vi "Line follower Color Stop.vi"(6 "Target reflection":sgl=25.0, 7 "Threshold to Color":i32=1200, 8 "Threshold to slow":i32=1000, 9 "Min. speed":i32=20, 10 "Max. speed":i32=40, 11 "EV3 in":T1) -> (3 "EV3 out":T1)   [LabVIEW 2016]
uses:
  <vilib>/NXT/Subs/LVHSConnector.ctl
  <vilib>/NXT/LegoClasses/BrickReference/BrickReference.lvclass
  <vilib>/NXT/Block Support/NXT_OutputPort.ctl
  <vilib>/NXT/Block Support/NXT_InputPort.ctl
  <vilib>/NXT/NXTIO Xnodes/NXTIONodeSubVIs/LEGOResetMotors.vi
  <vilib>/NXT/Dual Mode Library/Motors/Rotation.vi
  <vilib>/NXT/Dual Mode Library/Sensors/EV3_Color_Reflect.vi
  <vilib>/NXT/NXTIO Xnodes/NXTIONodeSubVIs/NXTMotorSteeringOn.vi
  <vilib>/NXT/NXTIO Xnodes/NXTIONodeSubVIs/NXTStopMotors.vi
  <vilib>/NXT/Dual Mode Library/Waits/Wait_Num.vi
  <vilib>/NXT/NXTIO Xnodes/NXTIOXNode/NXTIO.xnode
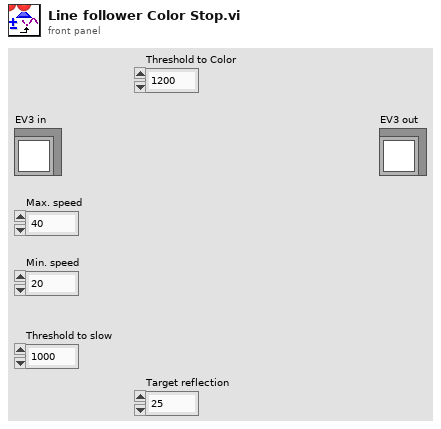
[diagram p1: front panel]
types:
  T1 = typedef "LVHSConnector.ctl" = refnum<class "BrickReference.lvclass">
  T2 = typedef "NXT_OutputPort.ctl" = u8
  T3 = typedef "NXT_InputPort.ctl" = u32
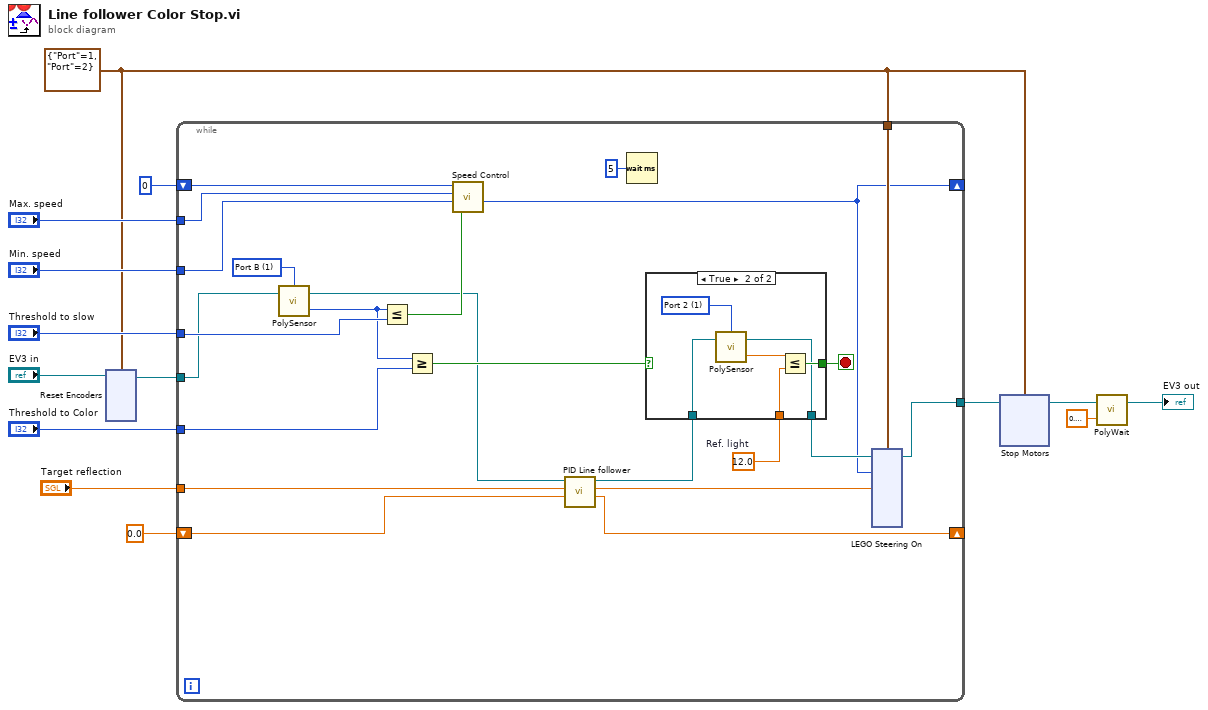
[diagram p0: block diagram]
diagram:
  w4 = cluster{"Port":T2, "Port":T2} {"Port"=1, "Port"=2} ("Motor")
  n1 = xnode "Reset Encoders"("Motors"=w4, "NXT/EV3"="EV3 in") -> ("NXT/EV3"=w10:T1)
  n2 = while {
    tunnel: w10 -> [w27]
    shift-right: [w37] -> _
    shift-left: sgl 0.0 -> [w24]
    tunnel: "Target reflection" -> [w36]
    tunnel: [w33] -> w6
    tunnel: w4 -> [w35]
    shift-right: [w17] -> _
    shift-left: 0 -> [w31]
    tunnel: "Min. speed" -> [w28]
    tunnel: "Max. speed" -> [w30]
    tunnel: "Threshold to slow" -> [w29]
    tunnel: "Threshold to Color" -> [w23]
    stop <- w22 stop-if-true
    w18 = sgl 12.0  # Ref. light
    w34 = T2 1 items=["Port A", "Port B", "Port C", "Port D"] ("Port (Port A)")
    n3 = call-poly <vilib>:"PolySensor.vi"("NXT/EV3"=w27, "Port (Port A)"=w34) -> ("Angle of Rotation"=w25:i32, "NXT/EV3"=w16:T1)  [unwired: 1 in]
    n4 = Less Or Equal?(x=w25, y=w29) -> (x <= y?=w26:bool)
    n5 = Greater Or Equal?(x=w25, y=w23) -> (x >= y?=w21:bool)
    n6 = call "Speed Control.vi"("Speed Up or Down?"=w26, "Min. speed"=w28, "Max. speed"=w30, "Ini. speed"=w31) -> ("Speed out"=w17:i32)  [unwired: 7 in]
    n7 = call "PID Line follower.vi"("Previous integral"=w24, "Target reflection"=w36, "EV3 in"=w16) -> ("New integral"=w37:sgl, "Total error"=w15:sgl, "EV3 out"=w20:T1)  [unwired: 5 in, 1 out]
    n8 = Wait (ms)(milliseconds to wait=u32 5) -> ()  [unwired: 1 out]
    n9 = case shown="True" w21 {
      tunnel: [_ w42] -> w22
      tunnel: w20 -> [w38 w41]
      tunnel: [w38 w40] -> w19
      tunnel: w18 -> [_ w39]
      frame False {
      }
      frame True {
        w44 = T3 1 items=["Port 1", "Port 2", "Port 3", "Port 4"] ("Port (Port 1)")
        n10 = call-poly <vilib>:"PolySensor.vi"("NXT/EV3"=w41, "Port (Port 1)"=w44) -> ("Scaled Value"=w43:sgl, "NXT/EV3"=w40:T1)  [unwired: 1 in]
        n11 = Less Or Equal?(x=w43, y=w39) -> (x <= y?=w42:bool)
      }
    }
    n12 = xnode "LEGO Steering On"("Steering 1"=w15, "Power 1"=w17, "Motors"=w35, "NXT/EV3"=w19) -> ("NXT/EV3"=w33:T1)
  }
  n13 = xnode "Stop Motors"("Motors"=w4, "NXT/EV3"=w6) -> ("NXT/EV3"=w5:T1)
  n14 = call-poly <vilib>:"PolyWait.vi"("Time (1 sec)"=sgl 0.2, "NXT/EV3"=w5) -> ("NXT/EV3"=→"EV3 out":T1)  [unwired: 2 in]
